vi "Consume Required Token.vi"(10 "Type":T2, 11 "Pattern Parser In":T3) -> (0 "error out":errorcluster, 2 "Token":T1, 3 "Pattern Parser":T3)   [LabVIEW 2020, in "Stream.lvlib" / "URLPattern.lvclass"]
uses:
  URLPattern.lvclass
  Pattern Parser.ctl
  Token.ctl
  Token Type.ctl
  Pattern Part.ctl
  Pattern Part Type.ctl
  Pattern Part Modifier.ctl
  Token Type Equals.vi
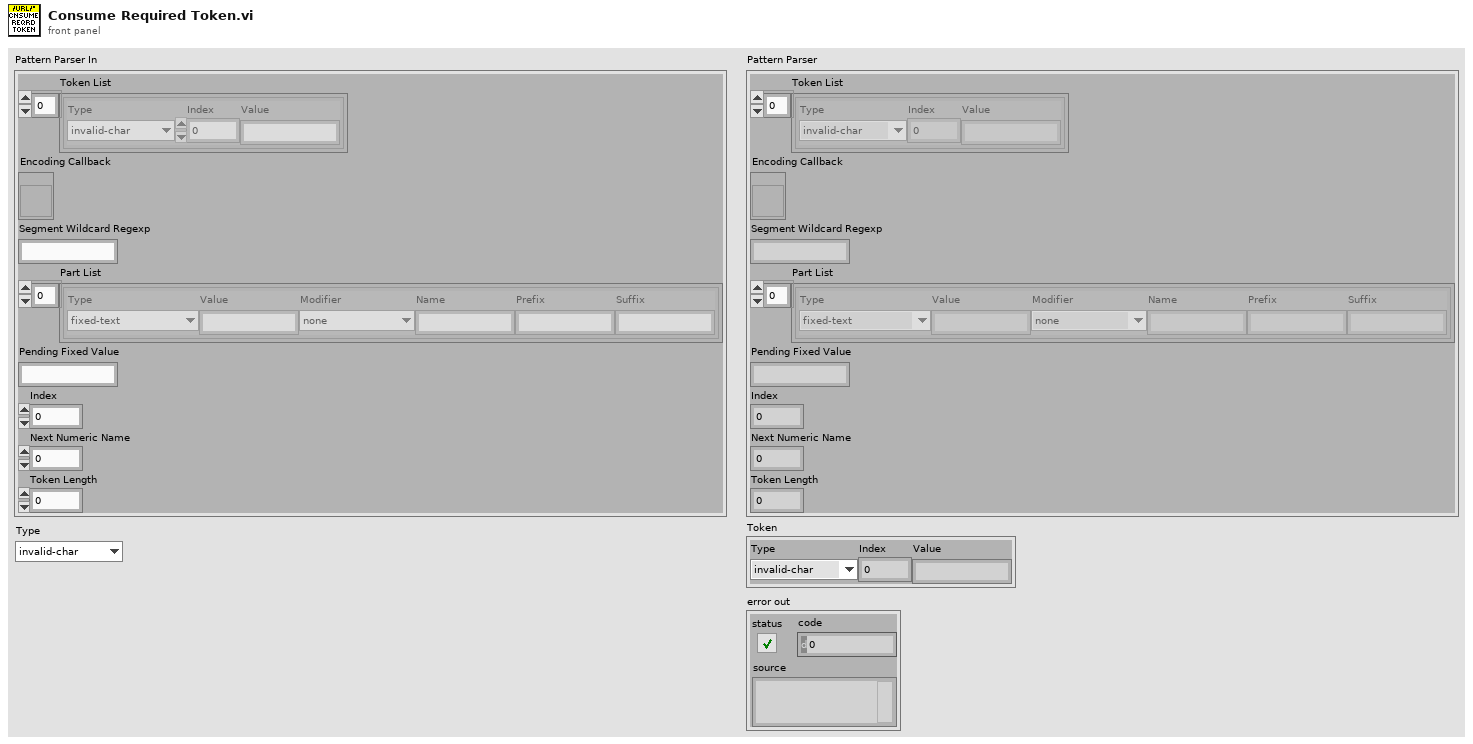
[diagram p1: front panel]
types:
  T1 = typedef "Stream.lvlib/URLPattern.lvclass/Token.ctl" = cluster{"Type":T2, "Index":i32, "Value":string}
  T2 = typedef "Stream.lvlib/URLPattern.lvclass/Token Type.ctl" = enum16{"invalid-char", "open", "close", "regexp", "name", "char", "escaped-char", "other-modifier", "asterisk", "end"}
  T3 = typedef "Stream.lvlib/URLPattern.lvclass/Pattern Parser.ctl" = cluster{"Token List":T1[], "Encoding Callback":refnum<vi>, "Segment Wildcard Regexp":string, "Part List":T4[], "Pending Fixed Value":string, "Index":i32, "Next Numeric Name":i32, "Token Length":i32}
  T4 = typedef "Stream.lvlib/URLPattern.lvclass/Pattern Part.ctl" = cluster{"Type":T5, "Value":string, "Modifier":T6, "Name":string, "Prefix":string, "Suffix":string}
  T5 = typedef "Stream.lvlib/URLPattern.lvclass/Pattern Part Type.ctl" = enum16{"fixed-text", "regexp", "segment-wildcard", "full-wildcard"}
  T6 = typedef "Stream.lvlib/URLPattern.lvclass/Pattern Part Modifier.ctl" = enum16{"none", "optional", "zero-or-more", "one-or-more"}
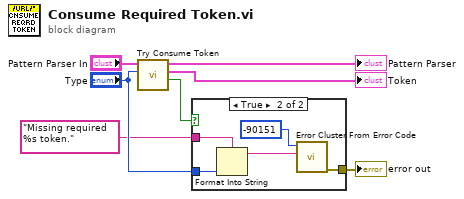
[diagram p0: block diagram]
diagram:
  n1 = call "Try Consume Token.vi"("Type"="Type", "Pattern Parser In"="Pattern Parser In") -> ("Null?"=w6:bool, "Token"=→"Token":T1, "Pattern Parser"=→"Pattern Parser":T3)  [unwired: 7 in]
  n2 = case shown="True" w6 {
    tunnel: "Type" -> [_ w12]
    tunnel: "Missing required %s token." -> [_ w10]
    tunnel: [_ w8] -> w1
    frame False {
    }
    frame True {
      n3 = Format Into String(format string=w10, w12) -> (resulting string=w9:string)  [unwired: 2 in, 1 out]
      n4 = call <vilib>:"Error Cluster From Error Code.vi"("error message (\"\")"=w9, "error code (0)"=-90151) -> ("error out"=w8:errorcluster)  [unwired: 7 in]
    }
  }
  "error out" <- w1
